vi "STOP.vi"(8 "error in (no error)":errorcluster, 11 "Stop in":refnum<class "UV-VIS_AVANTES.lvclass">) -> (0 "error out":errorcluster, 3 "Stop out":refnum<class "UV-VIS_AVANTES.lvclass">)   [LabVIEW 2020, in "UV-VIS_AVANTES.lvclass"]
uses:
  UV-VIS_AVANTES.lvclass
  C:/Dev/TRANCON/Classes/GeneralFunctionality/GeneralFunctionality.lvclass
  GeneralFunctionality/GeneralFunctionality.lvclass/GeneralFunctionality.ctl
  GeneralFunctionality/GeneralFunctionality.lvclass
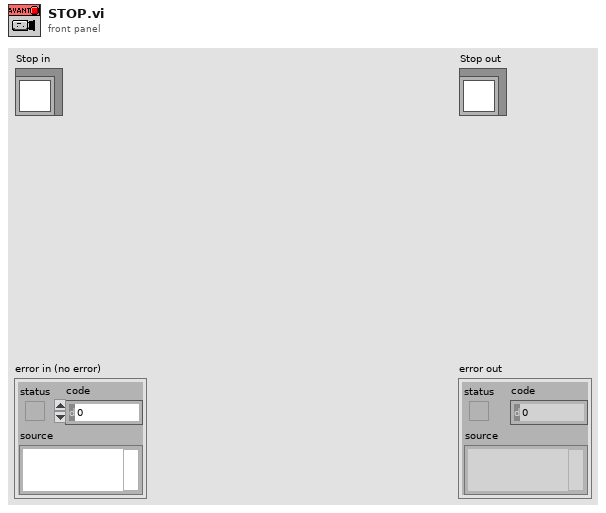
[diagram p1: front panel]
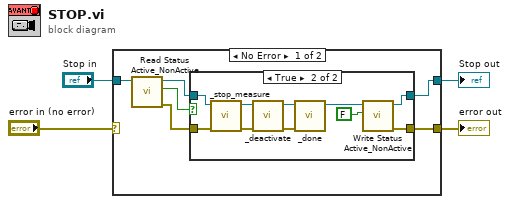
[diagram p0: block diagram]
diagram:
  n1 = case shown="No Error" "error in (no error)" {
    selector: "error in (no error)" -> [_ w23]
    tunnel: "Stop in" -> [w7 w24]
    tunnel: [w6 w24] -> w2
    tunnel: [w5 w23] -> w1
    frame No Error {
      n2 = call "Read Status Active_NonActive.vi"("GeneralFunctionality in"=w7) -> ("error out"=w8:errorcluster, "Status Active/NonActive"=w10:bool, "GeneralFunctionality out"=w9:refnum<class "UV-VIS_AVANTES.lvclass">)  [unwired: 8 in]
      n3 = case shown="True" w10 {
        tunnel: [w11 w21] -> w5
        tunnel: [w12 w22] -> w6
        tunnel: w9 -> [w12 w16]
        tunnel: w8 -> [w11 w19]
        frame False {
        }
        frame True {
          n4 = call "_stop_measure.vi"("error in (no error)"=w19, "UV-VIS_AVANTES in"=w16) -> ("error out"=w18:errorcluster, "UV-VIS_AVANTES out"=w17:refnum<class "UV-VIS_AVANTES.lvclass">)  [unwired: 8 in]
          n5 = call "_deactivate.vi"("error in (no error)"=w18, "UV-VIS_AVANTES in"=w17) -> ("error out"=w14:errorcluster, "UV-VIS_AVANTES out"=w15:refnum<class "UV-VIS_AVANTES.lvclass">)  [unwired: 8 in]
          n6 = call "_done.vi"("error in (no error)"=w14, "UV-VIS_AVANTES in"=w15) -> ("UV-VIS_AVANTES out"=w13:refnum<class "UV-VIS_AVANTES.lvclass">)  [unwired: 8 in, 1 out]
          n7 = call "Write Status Active_NonActive.vi"("Status Active/NonActive"=FALSE, "GeneralFunctionality in"=w13) -> ("error out"=w21:errorcluster, "GeneralFunctionality out"=w22:refnum<class "UV-VIS_AVANTES.lvclass">)  [unwired: 8 in]
        }
      }
    }
    frame Error {
    }
  }
  "error out" <- w1
  "Stop out" <- w2
